vi "analogowe - usun nieaktywne.vi"(6 "Kanaly aktywne":bool[](array[boolean]), 7 "#cores (1)":i32=1, 8 "error in (no error)":errorcluster, 10 "Kanaly in":T1) -> (0 "error out":errorcluster, 2 "Kanaly out":T1)   [LabVIEW 2013]
doc: "Usuwa nieaktywne kanały analogowe\nAktywnym nadaje numerację kanału oraz właściwość aktywny"
uses:
  Kontrolki/Przetwarzanie/Kanaly.ctl
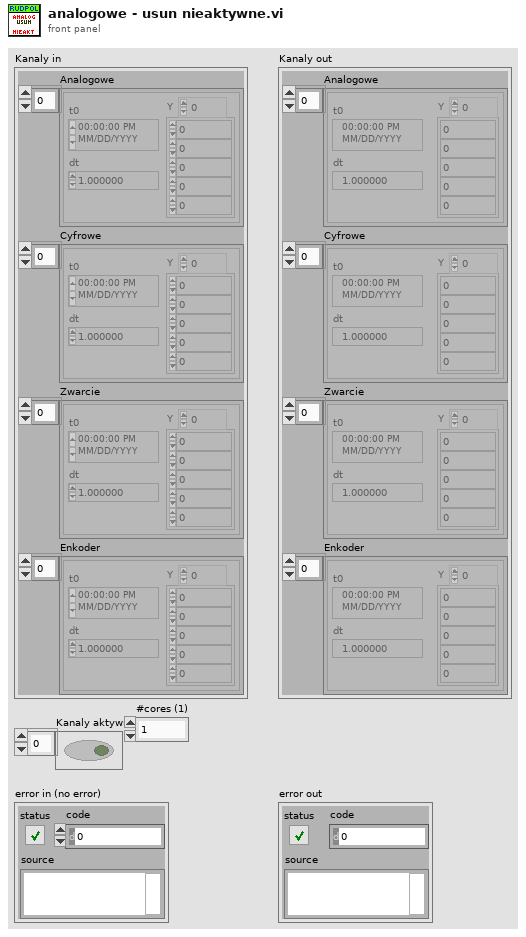
[diagram p1: front panel]
types:
  T1 = typedef "Kanaly.ctl" = cluster{"Analogowe":waveform(dbl)[], "Cyfrowe":waveform(dbl)[], "Zwarcie":waveform(dbl)[], "Enkoder":waveform(dbl)[]}
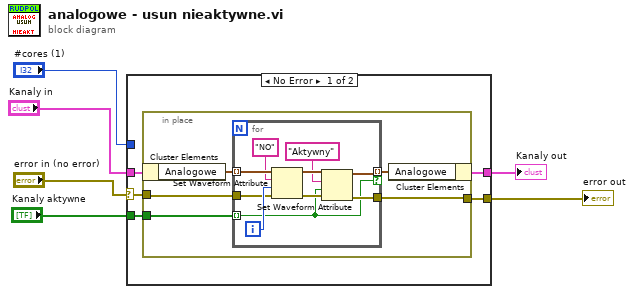
[diagram p0: block diagram]
diagram:
  n1 = case shown="No Error" "error in (no error)" {
    selector: "error in (no error)" -> [w7 w28]
    tunnel: [w11 w28] -> w6
    tunnel: "Kanaly aktywne" -> [w10 _]
    tunnel: [w9 w27] -> w4
    tunnel: "Kanaly in" -> [w8 w27]
    tunnel: "#cores (1)" -> [_ _]
    frame No Error {
      n2 = in-place {
        in-place-border: w10 -> [w14]
        in-place-border: w7 -> [w13]
        in-place-border: [w12] -> w11
        n3 = in-place-cluster #1(w8) -> ("Analogowe"=w16:waveform(dbl)[])
        n4 = for {
          tunnel: w16 -> [w26] mode=indexing
          tunnel: [w19] -> w15 mode=indexing if=w17
          tunnel: w14 -> [w17] mode=indexing
          tunnel: w13 -> [w23]
          tunnel: [w18] -> w12
          i -> [w25]
          n5 = Set Waveform Attribute(4:w23, 5:w25, 6:"NO", 7:w26) -> (0:w22:errorcluster, 3:w21:waveform(dbl))  [unwired: 1 out]
          n6 = Set Waveform Attribute(4:w22, 5:w17, 6:"Aktywny", 7:w21) -> (0:w18:errorcluster, 3:w19:waveform(dbl))  [unwired: 1 out]
        }
        n7 = in-place-cluster #1("Analogowe"=w15) -> (w9:T1)
      }
    }
    frame Error {
    }
  }
  "error out" <- w6
  "Kanaly out" <- w4
